vi "HexToNormalString.vi"(7 "Hex Display":string="\u0001") -> (8 "Normal Display":string)   [LabVIEW 2014]
doc: "This VI translate the hex display string to normal display string. The two type string display the same."
panel:
  out "数值":i32
  out "无符号字节数组":u8[](array[numeric])
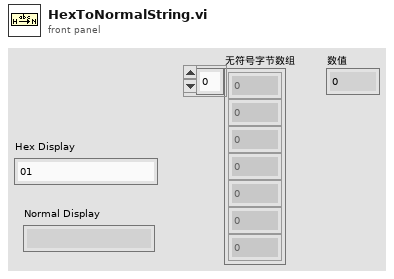
[diagram p1: front panel]
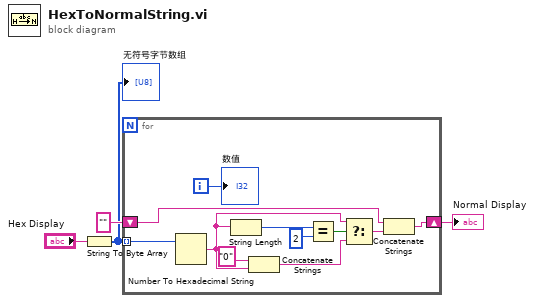
[diagram p0: block diagram]
diagram:
  n1 = String To Byte Array(string="Hex Display") -> (unsigned byte array=w2:u8[])
  "无符号字节数组" <- w2
  n2 = for {
    tunnel: w2 -> [w15] mode=indexing
    shift-right: [w14] -> w3
    shift-left: "" -> [w13]
    i -> [w5]
    n3 = Number To Hexadecimal String(2:w15) -> (0:w8:string)  [unwired: 1 in]
    n4 = String Length(string=w8) -> (length=w12:i32)
    n5 = Concatenate Strings("0" ("字符串"), w8) -> (w6:string)
    n6 = Equal?(x=w12, y=2) -> (x = y?=w10:bool)
    n7 = Select(t=w8, s=w10, f=w6) -> (s? t:f=w9:string)
    n8 = Concatenate Strings(w13, w9) -> (w14:string)
    "数值" <- w5
  }
  "Normal Display" <- w3
